vi "17.Evd.6_Ask.3.vi"() -> ()   [LabVIEW 2025]
panel:
  out "C":dbl[][](array[numeric])
  out "A":dbl[][](array[numeric])
  out "D = A + 1":dbl[][](array[numeric])
  out "B":dbl[][](array[numeric])
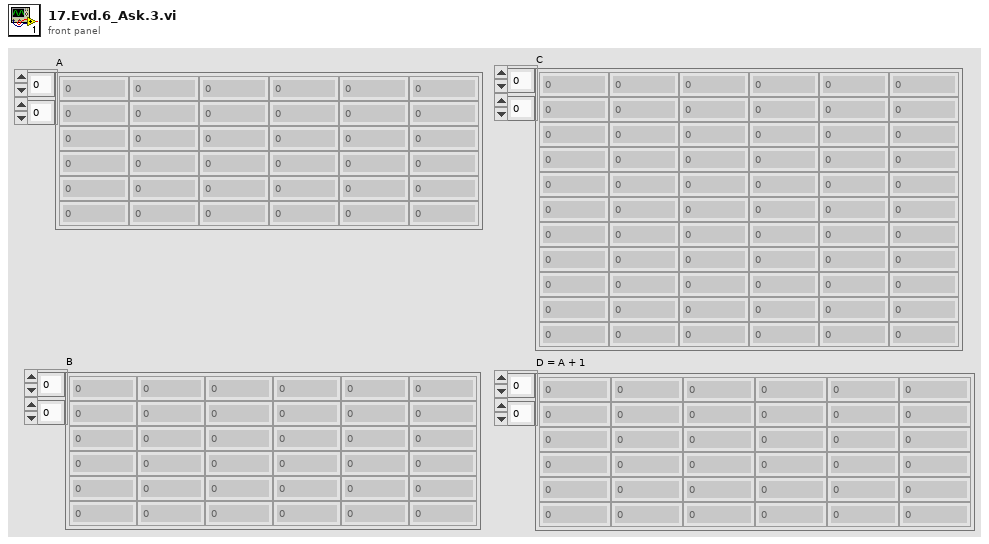
[diagram p1: front panel]
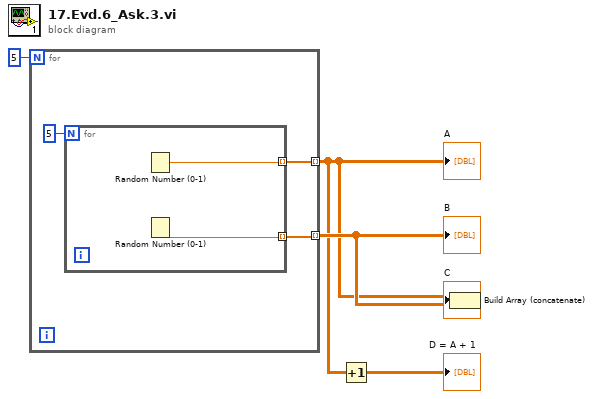
[diagram p0: block diagram]
diagram:
  n1 = for {
    N: 5 -> [_]
    tunnel: [w7] -> w2 mode=indexing
    tunnel: [w6] -> w4 mode=indexing
    n2 = for {
      N: 5 -> [_]
      tunnel: [w10] -> w7 mode=indexing
      tunnel: [w9] -> w6 mode=indexing
      n3 = Random Number (0-1)() -> (number: 0 to 1=w10:dbl)
      n4 = Random Number (0-1)() -> (number: 0 to 1=w9:dbl)
    }
  }
  "B" <- w4
  "A" <- w2
  n5 = Increment(x=w2) -> (x+1=→"D = A + 1":dbl[][])
  n6 = Build Array (concatenate)(w2, w4) -> (→"C":dbl[][])
